vi "Write Gain Values to Default.vi"(6 "error in":errorcluster, 8 "MaxRead":i32, 9 "Channel in":u16) -> (0 "error out":errorcluster, 1 "Messages":T1(array[cluster]), 2 "Pass":bool, 3 "Channel out":u16)   [LabVIEW 2023]
uses:
  4f930f32-d09a-43ef-bca1-8b214b378bd5.vi
  e8470de1-fa2d-4ee3-b50e-96bd89dc731f.vi
  Communication/PCAN2023/PCAN API.lvlib
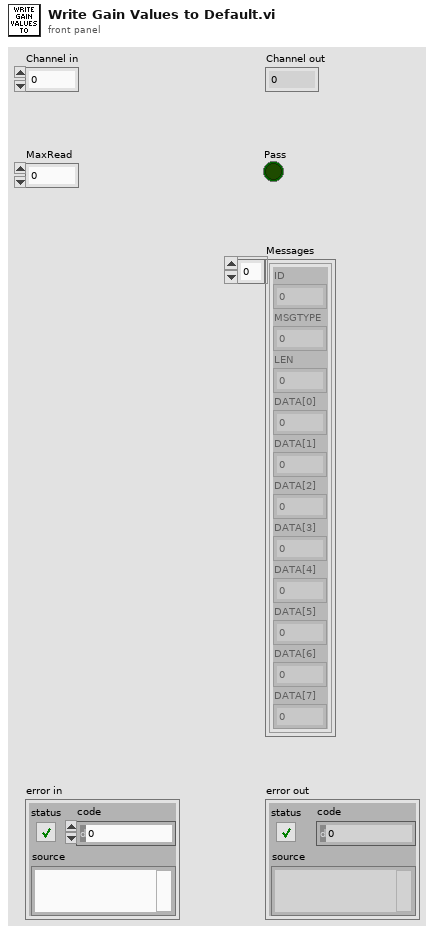
[diagram p1: front panel]
types:
  T1 = cluster{"ID":u32, "MSGTYPE":u8, "LEN":u8, "DATA[0]":u8, "DATA[1]":u8, "DATA[2]":u8, "DATA[3]":u8, "DATA[4]":u8, "DATA[5]":u8, "DATA[6]":u8, "DATA[7]":u8}[]
  T2 = cluster{"ID":u32, "MSGTYPE":u8, "LEN":u8, "DATA[0]":u8, "DATA[1]":u8, "DATA[2]":u8, "DATA[3]":u8, "DATA[4]":u8, "DATA[5]":u8, "DATA[6]":u8, "DATA[7]":u8}
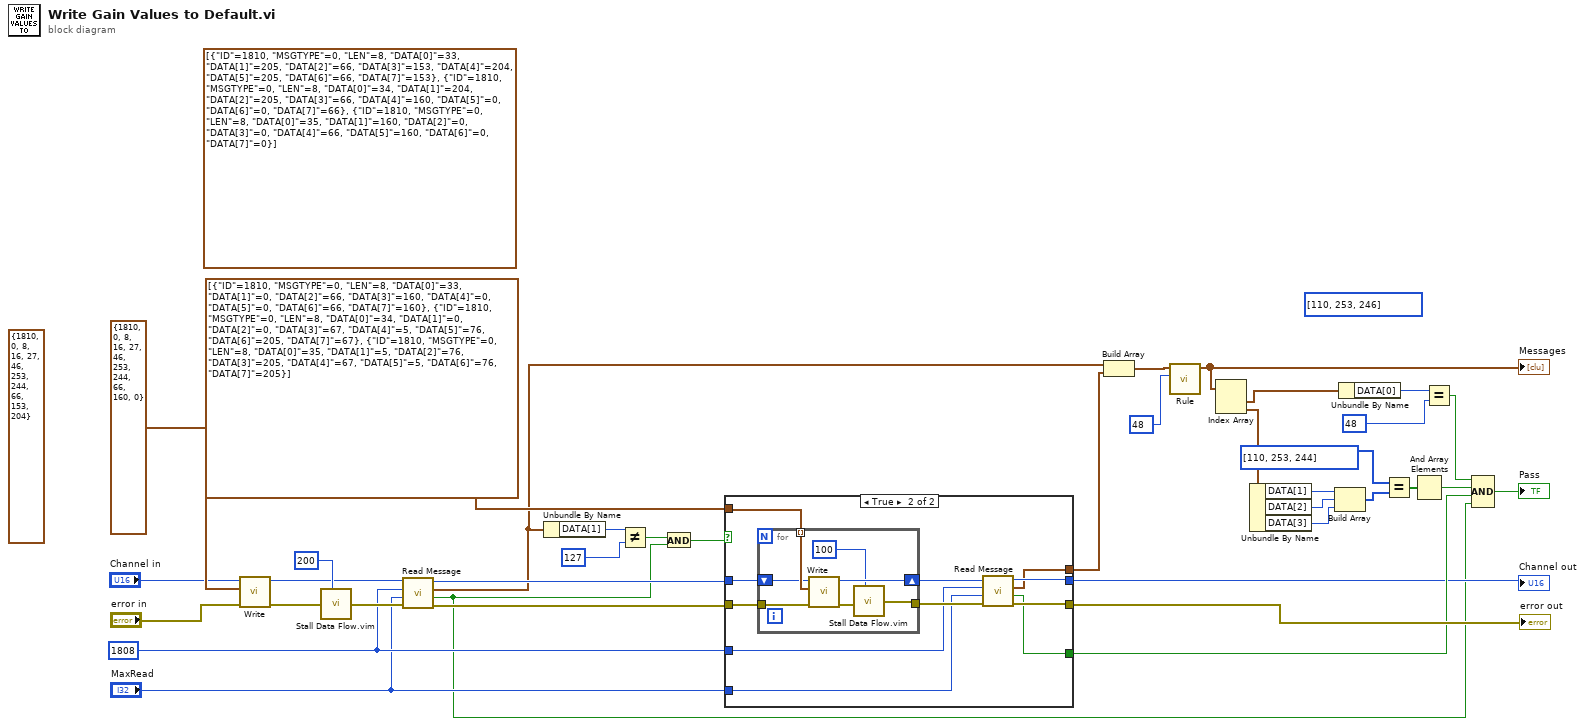
[diagram p0: block diagram]
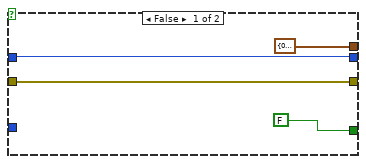
[diagram p2: hidden frame]
diagram:
  (unwired) T1 [{"ID"=1810, "MSGTYPE"=0, "LEN"=8, "DATA[0]"=33, "DATA[1]"=205, "DATA[2]"=66, "DATA[3]"=153, "DATA[4]"=204, "DATA[5]"=205, "DATA[6]"=66, "DATA[7]"=153}, {"ID"=1810, "MSGTYPE"=0, "LEN"=8, "DATA[0]"=34, "DATA[1]"=204, "DATA[2]"=205, "DATA[3]"=66, "DATA[4]"=160, "DATA[5]"=0, "DATA[6]"=0, "DATA[7]"=66}, {"ID"=1810, "MSGTYPE"=0, "LEN"=8, "DATA[0]"=35, "DATA[1]"=160, "DATA[2]"=0, "DATA[3]"=0, "DATA[4]"=66, "DATA[5]"=160, "DATA[6]"=0, "DATA[7]"=0}] ("MessageBuffer")
  (unwired) T2 {"ID"=1810, "MSGTYPE"=0, "LEN"=8, "DATA[0]"=16, "DATA[1]"=27, "DATA[2]"=46, "DATA[3]"=253, "DATA[4]"=244, "DATA[5]"=66, "DATA[6]"=153, "DATA[7]"=204} ("MessageBuffer")
  (unwired) u8[] [110, 253, 246] ("x")
  (unwired) u32 200 ("milliseconds to wait")
  w10 = u32 1808 ("ID")
  n1 = call "Write.vi"("error in"="error in", "MessageBuffer"=T2 {"ID"=1810, "MSGTYPE"=0, "LEN"=8, "DATA[0]"=16, "DATA[1]"=27, "DATA[2]"=46, "DATA[3]"=253, "DATA[4]"=244, "DATA[5]"=66, "DATA[6]"=160, "DATA[7]"=0}, "Channel"="Channel in") -> ("error out"=w25:errorcluster, "Channel out"=w15:u16)  [unwired: 5 in, 2 out]
  n2 = call "Stall Data Flow.vim"("value in"=w25, "milliseconds to wait"=u32 200) -> ("value out"=w13:errorcluster)  [unwired: 1 out]
  n3 = call "Read Message.vi"("error in"=w13, "MaxRead"="MaxRead", "ID"=w10, "Channel in"=w15) -> ("error out"=w12:errorcluster, "Passed"=w6:bool, "Last Message"=w11:T2, "Channel out"=w14:u16)  [unwired: 3 in, 1 out]
  n4 = Unbundle By Name(w11) -> ("DATA[1]"=w16:u8)
  n5 = Not Equal?(x=w16, y=u8 127) -> (x != y?=w8:bool)
  n6 = And(x=w8, y=w6) -> (x .and. y?=w7:bool)
  n7 = case shown="True" w7 {
    tunnel: T1 [{"ID"=1810, "MSGTYPE"=0, "LEN"=8, "DATA[0]"=33, "DATA[1]"=0, "DATA[2]"=66, "DATA[3]"=160, "DATA[4]"=0, "DATA[5]"=0, "DATA[6]"=66, "DATA[7]"=160}, {"ID"=1810, "MSGTYPE"=0, "LEN"=8, "DATA[0]"=34, "DATA[1]"=0, "DATA[2]"=0, "DATA[3]"=67, "DATA[4]"=5, "DATA[5]"=76, "DATA[6]"=205, "DATA[7]"=67}, {"ID"=1810, "MSGTYPE"=0, "LEN"=8, "DATA[0]"=35, "DATA[1]"=5, "DATA[2]"=76, "DATA[3]"=205, "DATA[4]"=67, "DATA[5]"=5, "DATA[6]"=76, "DATA[7]"=205}] ("MessageBuffer") -> [_ w53]
    tunnel: w14 -> [w41 w52]
    tunnel: w12 -> [w40 w51]
    tunnel: [w40 w47] -> w21
    tunnel: [FALSE w43] -> w20
    tunnel: [w41 w48] -> w19
    tunnel: [T2 {"ID"=0, "MSGTYPE"=0, "LEN"=0, "DATA[0]"=0, "DATA[1]"=0, "DATA[2]"=0, "DATA[3]"=0, "DATA[4]"=0, "DATA[5]"=0, "DATA[6]"=0, "DATA[7]"=0} ("MessageBuffer out") w46] -> w18
    tunnel: w10 -> [_ w45]
    tunnel: "MaxRead" -> [_ w44]
    frame False {
    }
    frame True {
      n8 = for {
        tunnel: w53 -> [w60] mode=indexing
        shift-right: [w57] -> w50
        shift-left: w52 -> [w59]
        tunnel: w51 -> [w58]
        tunnel: [w54] -> w49
        n9 = call "Write.vi"("error in"=w58, "MessageBuffer"=w60, "Channel"=w59) -> ("error out"=w55:errorcluster, "Channel out"=w57:u16)  [unwired: 5 in, 2 out]
        n10 = call "Stall Data Flow.vim"("value in"=w55, "milliseconds to wait"=u32 100) -> ("value out"=w54:errorcluster)  [unwired: 1 out]
      }
      n11 = call "Read Message.vi"("error in"=w49, "MaxRead"=w44, "ID"=w45, "Channel in"=w50) -> ("error out"=w47:errorcluster, "Passed"=w43:bool, "Last Message"=w46:T2, "Channel out"=w48:u16)  [unwired: 3 in, 1 out]
    }
  }
  "error out" <- w21
  "Channel out" <- w19
  n12 = Build Array(w11, w18) -> (w5:T1)
  n13 = call "Rule.vi"("Case"=u8 48 ("y"), "Array in"=w5) -> ("Array out"=w3:T1)  [unwired: 9 in]
  "Messages" <- w3
  n14 = Index Array(array=w3) -> (element #1=w2:T2, element #2=w1:T2)  [unwired: 2 in]
  n15 = Unbundle By Name(w1) -> ("DATA[1]"=w32:u8, "DATA[2]"=w31:u8, "DATA[3]"=w30:u8)
  n16 = Build Array(w32, w31, w30) -> (w29:u8[])
  n17 = Unbundle By Name(w2) -> ("DATA[0]"=w24:u8)
  n18 = Equal?(x=u8[] [110, 253, 244], y=w29) -> (x = y?=w34:bool[])
  n19 = And Array Elements(Boolean array=w34) -> (logical AND=w28:bool)
  n20 = Equal?(x=w24, y=u8 48) -> (x = y?=w22:bool)
  n21 = Compound Arithmetic op=AND(w22, w28, w20, w6) -> (→"Pass":bool)
